vi "Get DAQ Analog Data Value.vi"(0 "DAQ":refnum<class "DAQ.lvclass">, 5 "IOName (enum)":variant, 9 "Name":string, 11 "error in (no error)":errorcluster, 12 "Raw? (false)":bool) -> (4 "DAQ":refnum<class "DAQ.lvclass">, 8 "Value":dbl, 15 "error out":errorcluster)   [LabVIEW 2017, in "DAQ.lvclass"]
doc: "Developed by Kevin Thompson\nkevin@thompsonengineering.net\n\nCopyright 2018-2020\nThompson Engineering, LLC"
uses:
  DAQ.lvclass
  DAQ.lvclass/DAQ.ctl
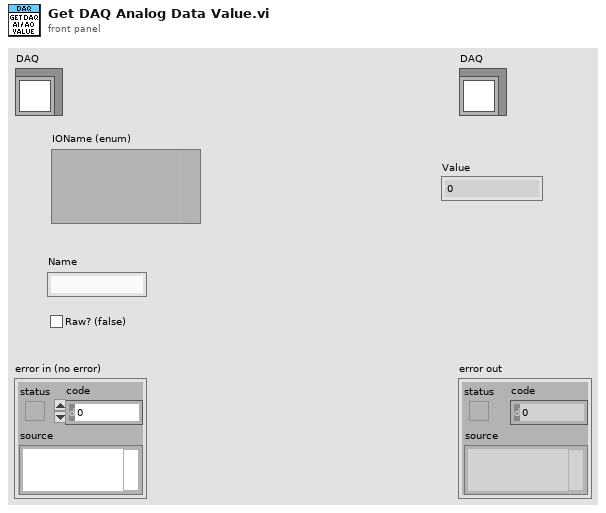
[diagram p1: front panel]
types:
  T1 = typedef "Type Descriptor Enumeration__ogtk.ctl" = enum8{"<Null>", "I8", "I16", "I32", "I64", "U8", "U16", "U32", "U64", "SGL", "DBL", "EXT", "CSG", "CDB", "CXT", "0x0F", "0x10", "0x11", "0x12", "0x13", "0x14", "Enum U8", "Enum U16", "Enum U32", "Enum U64", "SGL PQ", "DBL PQ", "EXT PQ", "CSG PQ", "CDB PQ", "CXT PQ", "0x1F", "0x20", "Boolean", "0x22", "0x23", "0x24", "0x25", "0x26", "0x27", "0x28", "0x29", "0x2A", "0x2B", "0x2C", "0x2D", "0x2E", "0x2F", "String", "0x31", "Path", "Pict", "0x34", "0x35", "0x36", "DAQ", "0x38", "0x39", "0x3A", "0x3B", "0x3C", "0x3D", "0x3E", "0x3F", "Array", "0x41", "0x42", "0x43", "0x44", "0x45", "0x46", "0x47", "0x48", "0x49", "0x4A", "0x4B", "0x4C", "0x4D", "0x4E", "0x4F", "Cluster", "0x51", "0x52", "Variant", "Waveform", "0x55", "0x56", "0x57", "0x58", "0x59", "0x5A", "0x5B", "0x5C", "0x5D", "0x5E", "0x5F", "0x60", "0x61", "0x62", "0x63", "0x64", "0x65", "0x66", "0x67", "0x68", "0x69", "0x6A", "0x6B", "0x6C", "0x6D", "0x6E", "0x6F", "Refnum"}
  T2 = typedef "TD Dynamic CVT DVR--ref.ctl" = refnum<data-value>
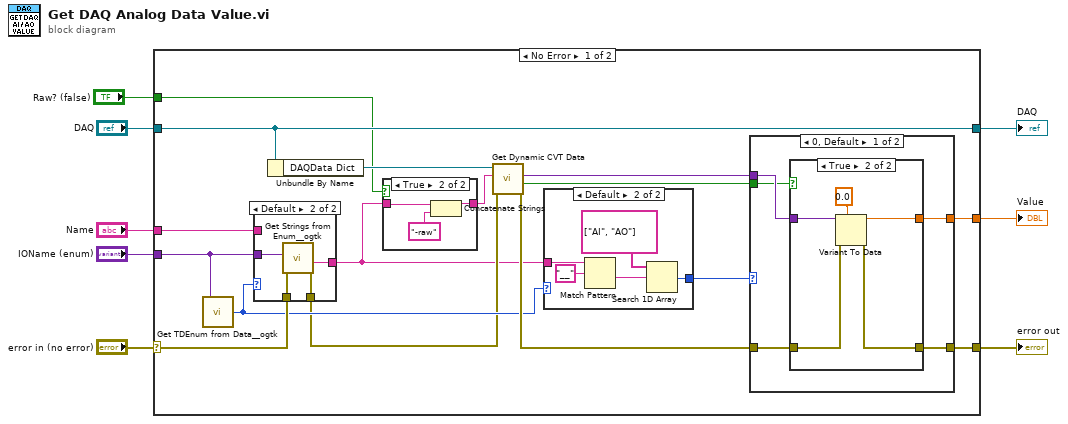
[diagram p0: block diagram]
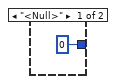
[diagram p4: hidden frame]
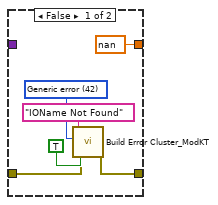
[diagram p5: hidden frame]
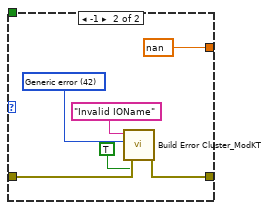
[diagram p6: hidden frame]
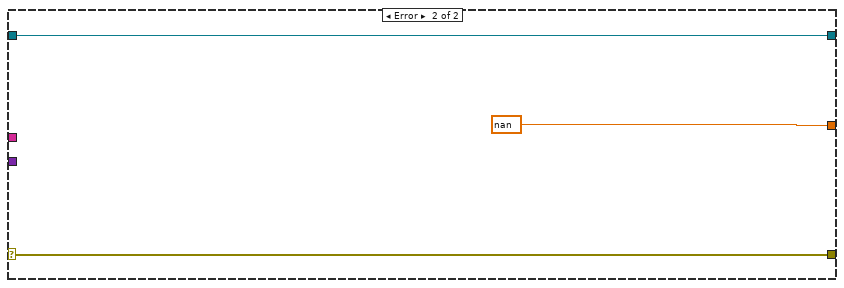
[diagram p7: hidden frame]
diagram:
  n1 = case shown="No Error" "error in (no error)" {
    selector: "error in (no error)" -> [w24 w65]
    tunnel: [w19 w65] -> w7
    tunnel: [w23 w64] -> w5
    tunnel: "DAQ" -> [w23 w64]
    tunnel: "IOName (enum)" -> [w15 _]
    tunnel: [w16 nan] -> w3
    tunnel: "Name" -> [w13 _]
    tunnel: "Raw? (false)" -> [w11 _]
    frame No Error {
      n2 = call <userlib>:"Get TDEnum from Data__ogtk.vi"("Data"=w15) -> ("Type Descriptor Enumeration"=w14:T1)  [unwired: 4 in]
      n3 = case shown="Default" w14 {
        tunnel: w15 -> [_ w34]
        tunnel: w24 -> [w29 w33]
        tunnel: [w30 w32] -> w10
        tunnel: w13 -> [w30 _]
        tunnel: [w29 w31] -> w12
        frame "<Null>" {
        }
        frame Default {
          n4 = call <userlib>:"Get Strings from Enum__ogtk.vi"("error in (no error)"=w33, "Enum"=w34) -> ("error out"=w31:errorcluster, "String Value"=w32:string)  [unwired: 6 in, 2 out]
        }
      }
      n5 = Unbundle By Name(w23) -> ("DAQData Dict"=w22:T2)
      n6 = case shown="True" w11 {
        tunnel: w10 -> [w25 w27]
        tunnel: [w25 w28] -> w9
        frame False {
        }
        frame True {
          n7 = Concatenate Strings(w27, "-raw" ("string")) -> (w28:string)
        }
      }
      n8 = call <vilib>:"Get Dynamic CVT Data.vi"("error in (no error)"=w12, "DataName"=w9, "dCVT DVR"=w22) -> ("error out"=w21:errorcluster, "found"=w17:bool, "value"=w18:variant)  [unwired: 5 in, 1 out]
      n9 = case shown="Default" w14 {
        tunnel: w10 -> [_ w40]
        tunnel: [0 ("index of element") w36] -> w20
        frame "<Null>" {
        }
        frame Default {
          n10 = Match Pattern(string=w40, regular expression="__") -> (after substring=w38:string)  [unwired: 1 in, 3 out]
          n11 = Search 1D Array(1D array=string[] ["AI", "AO"], element=w38) -> (index of element=w36:i32)  [unwired: 1 in]
        }
      }
      n12 = case shown="0, Default" w20 {
        tunnel: w21 -> [w45 w61]
        tunnel: [w44 w62] -> w19
        tunnel: w18 -> [w43 _]
        tunnel: w17 -> [w41 _]
        tunnel: [w42 nan] -> w16
        frame 0, Default {
          n13 = case shown="True" w41 {
            tunnel: w45 -> [w48 w56]
            tunnel: [w47 w55] -> w44
            tunnel: w43 -> [_ w54]
            tunnel: [nan w52] -> w42
            frame False {
              w50 = 42 items=["No error", "Argument error", "Memory is full", "Out of zone", "End of file", "File already open", "Generic file I/O error", "File not found", "File permission error", "Disk is full", "Duplicate path", "Too many files open", "System feature not enabled", "Resource file not found", "Cannot add resource", "Resource not found", "Image not found", "Image memory error", "Pen does not exist", "Config type invalid", "Config token not found", "Config parse error", "Config memory error", "Bad external code format", "Bad external code offset", "External code not present", "Null window", "Destroy window error", "Null menu", "Print aborted", "Bad print record", "Print driver error", "Windows error during printing", "Memory error during printing", "Print dialog error", "Generic print error", "Invalid device refnum", "Device not found", "Device parameter error", "Device unit error", "Cannot open device", "Device call aborted", "Generic error", "Cancelled by user", "Object ID too low", "Object ID too high", "Object not in heap", "Unknown heap", "Unknown object (invalid DefProc)", "Unknown object (DefProc not in table)", "Message out of range", "Invalid (null) method", "Unknown message", "Manager call not supported", "Bad address", "Network operation in progress", "Network operation timed out", "Connection is busy", "Network attribute not supported", "Network error", "Address in use", "System out of memory", "Connection aborted", "Connection refused", "Not connected", "Already connected", "Connection closed", "Initialization error (interapplication manager)", "Bad occurrence", "Wait on unbound occurrence handler", "Occurrence queue overflow", "Datalog type conflict", "Unused", "Unrecognized type (interapplication manager)", "Memory corrupt", "Failed to make temporary DLL", "Old CIN version", "Drag socket not found", "Failed to load drop-object", "Failed to register OLE object", "Failed to release OLE object", "Format specifier type mismatch", "Unknown format specifier", "Too few format specifiers", "Too many format specifiers", "Scan failed", "Newer CIN version", "Error converting to variant", "Runtime menu error", "Password tampered", "Variant attribute not found", "Incompatible variant data type", "Event data is not available", "Event Store is not present", "Occurrence is not found", "Event Queue is not created", "Event info is not available", "Refnum passed is NULL", "Error retrieving Class GUID", "Error retrieving CoClass GUID", "Error retrieving TypeLib GUID.", "Bad built application magic bytes.", "Specific driver is different from the specific driver associated with the Logical Name.", "There is no session opened to the class driver.", "Max Error", "MAX - Error with config objects", "MAX - Error loading configuration", "MAX - Group not supported"]
              n14 = call <vilib>:"Build Error Cluster_ModKT .vi"("Prepend String (\"\")"="IOName Not Found" ("Prepend String (\"\")"), "code"=w50, "error? (F)"=TRUE, "error in (no error)"=w48) -> ("error out"=w47:errorcluster)  [unwired: 3 in, 1 out]
            }
            frame True {
              n15 = Variant To Data(error in=w56, type=0.0, Variant=w54) -> (data=w52:dbl, error out=w55:errorcluster)
            }
          }
        }
        frame -1 {
          w59 = 42 items=["No error", "Argument error", "Memory is full", "Out of zone", "End of file", "File already open", "Generic file I/O error", "File not found", "File permission error", "Disk is full", "Duplicate path", "Too many files open", "System feature not enabled", "Resource file not found", "Cannot add resource", "Resource not found", "Image not found", "Image memory error", "Pen does not exist", "Config type invalid", "Config token not found", "Config parse error", "Config memory error", "Bad external code format", "Bad external code offset", "External code not present", "Null window", "Destroy window error", "Null menu", "Print aborted", "Bad print record", "Print driver error", "Windows error during printing", "Memory error during printing", "Print dialog error", "Generic print error", "Invalid device refnum", "Device not found", "Device parameter error", "Device unit error", "Cannot open device", "Device call aborted", "Generic error", "Cancelled by user", "Object ID too low", "Object ID too high", "Object not in heap", "Unknown heap", "Unknown object (invalid DefProc)", "Unknown object (DefProc not in table)", "Message out of range", "Invalid (null) method", "Unknown message", "Manager call not supported", "Bad address", "Network operation in progress", "Network operation timed out", "Connection is busy", "Network attribute not supported", "Network error", "Address in use", "System out of memory", "Connection aborted", "Connection refused", "Not connected", "Already connected", "Connection closed", "Initialization error (interapplication manager)", "Bad occurrence", "Wait on unbound occurrence handler", "Occurrence queue overflow", "Datalog type conflict", "Unused", "Unrecognized type (interapplication manager)", "Memory corrupt", "Failed to make temporary DLL", "Old CIN version", "Drag socket not found", "Failed to load drop-object", "Failed to register OLE object", "Failed to release OLE object", "Format specifier type mismatch", "Unknown format specifier", "Too few format specifiers", "Too many format specifiers", "Scan failed", "Newer CIN version", "Error converting to variant", "Runtime menu error", "Password tampered", "Variant attribute not found", "Incompatible variant data type", "Event data is not available", "Event Store is not present", "Occurrence is not found", "Event Queue is not created", "Event info is not available", "Refnum passed is NULL", "Error retrieving Class GUID", "Error retrieving CoClass GUID", "Error retrieving TypeLib GUID.", "Bad built application magic bytes.", "Specific driver is different from the specific driver associated with the Logical Name.", "There is no session opened to the class driver.", "Max Error", "MAX - Error with config objects", "MAX - Error loading configuration", "MAX - Group not supported"]
          n16 = call <vilib>:"Build Error Cluster_ModKT .vi"("Prepend String (\"\")"="Invalid IOName" ("Prepend String (\"\")"), "code"=w59, "error? (F)"=TRUE, "error in (no error)"=w61) -> ("error out"=w62:errorcluster)  [unwired: 3 in, 1 out]
        }
      }
    }
    frame Error {
    }
  }
  "error out" <- w7
  "DAQ" <- w5
  "Value" <- w3
